vi "GLdrv_PUL_RPMC.vi"(0 "Connection ID":T1, 5 "CH":i32=1 min=1, 7 "PRM Count":i32, 11 "error in (no error)":errorcluster, 13 "Query(f)":bool) -> (4 "Connection ID Out":T1, 8 "PRM Count out":i32, 15 "error out":errorcluster)   [LabVIEW 2017, in "GL860_Driver.lvlib"]
doc: "1回転のパルス数の設定・参照\nFUNCtionがREVO（回転数）の時に有効な機能です。\n指定したパルス数を１回転とします\n例）　設定値が10で入力が100カウントの時→ 回転数＝10\n設定値が16で入力が4569カウントの時→ 回転数＝285\n例）　:PUL:CH1:RPMC 360 (パルスCH1の１回転のパルス数を\n360パルスに設定します)"
uses:
  GL860_Driver.lvlib
  ConnectionID.ctl
  GLdrv_RW.ctl
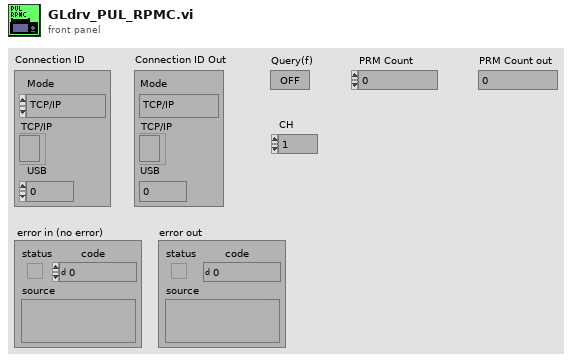
[diagram p1: front panel]
types:
  T1 = typedef "ConnectionID.ctl" = cluster{"Mode":enum16{"TCP/IP", "USB"}, "TCP/IP":refnum<k5>, "USB":i32}
  T2 = typedef "GLdrv_RW.ctl" = enum16{"Auto", "Read", "Write", "Buffer"}
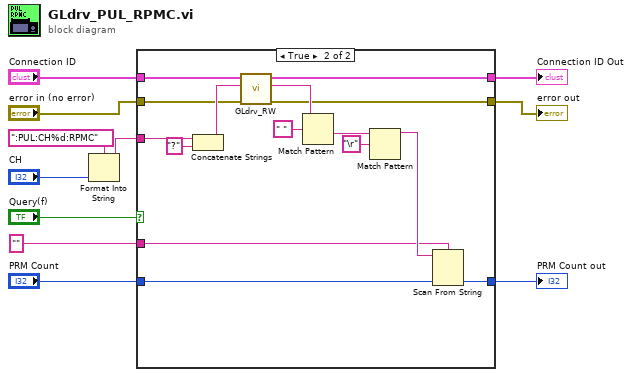
[diagram p0: block diagram]
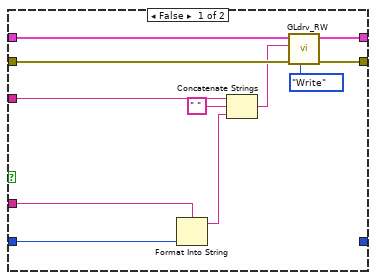
[diagram p2: hidden frame]
diagram:
  n1 = Format Into String(format string=":PUL:CH%d:RPMC" ("Command"), "CH") -> (resulting string=w5:string)  [unwired: 2 in, 1 out]
  n2 = case shown="TRUE" "Query(f)" {
    tunnel: w5 -> [w22 w34]
    tunnel: [w17 w26] -> w11
    tunnel: [w19 w30] -> w10
    tunnel: "Connection ID" -> [w20 w31]
    tunnel: "error in (no error)" -> [w18 w27]
    tunnel: "PRM Count" -> [w13 w25]
    tunnel: [_ w24] -> w2
    tunnel: "" ("Param") -> [w12 w23]
    frame False {
      n3 = Format Into String(format string=w12, w13) -> (resulting string=w14:string)  [unwired: 2 in, 1 out]
      n4 = Concatenate Strings(w22, " " ("string"), w14) -> (w16:string)
      n5 = call "GLdrv_RW.vi"("Mode(read)"=GLdrv_RW."Write", "error in (no error)"=w18, "data in"=w16, "Connection ID"=w20) -> ("error out"=w17:errorcluster, "Connection ID Out"=w19:T1)  [unwired: 3 in, 3 out]
    }
    frame True {
      n6 = Concatenate Strings(w34, "?" ("string")) -> (w29:string)
      n7 = call "GLdrv_RW.vi"("error in (no error)"=w27, "data in"=w29, "Connection ID"=w31) -> ("error out"=w26:errorcluster, "data out"=w28:string, "Connection ID Out"=w30:T1)  [unwired: 4 in, 2 out]
      n8 = Match Pattern(string=w28, regular expression=" " ("search string/char (-)")) -> (after substring=w35:string)  [unwired: 4 out]
      n9 = Match Pattern(string=w35, regular expression="\r") -> (before substring=w32:string)  [unwired: 4 out]
      n10 = Scan From String(format string=w23, input string=w32, default 1=w25) -> (output 1=w24:i32)  [unwired: 2 in, 3 out]
    }
  }
  "Connection ID Out" <- w10
  "error out" <- w11
  "PRM Count out" <- w2
